vi "题目6.vi"() -> ()   [LabVIEW 2017]
panel:
  out "平均值":dbl
  out "最小值":dbl
  out "最大值":dbl
  out "波形图":dbl[](graph)
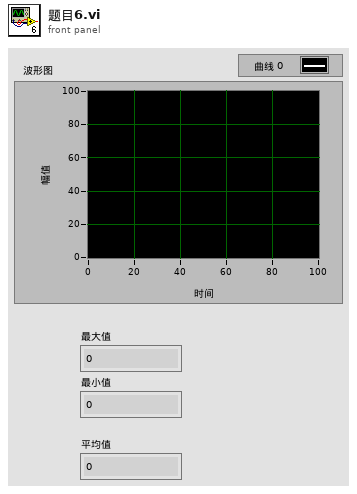
[diagram p1: front panel]
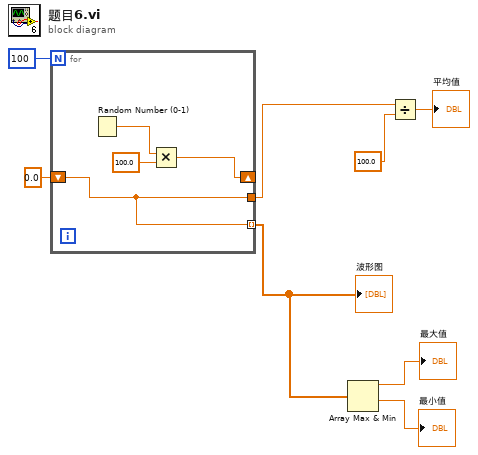
[diagram p0: block diagram]
diagram:
  n1 = for {
    N: 100 -> [_]
    shift-right: [w10] -> _
    shift-left: 0.0 -> [w9]
    tunnel: [w9] -> w3
    tunnel: [w9] -> w1 mode=indexing
    n2 = Random Number (0-1)() -> (number: 0 to 1=w12:dbl)
    n3 = Multiply(x=w12, y=100.0) -> (x*y=w10:dbl)
  }
  "波形图" <- w1
  n4 = Array Max & Min(array=w1) -> (max value=→"最大值":dbl, min value=→"最小值":dbl)  [unwired: 2 out]
  n5 = Divide(x=w3, y=100.0) -> (x/y=→"平均值":dbl)
